vi "ABB clear results.vi"   [LabVIEW 2017]
uses:
  ABB global.vi
panel:
  # "clear tests"
types:
  T1 = cluster{"Stator R":dbl, "Stator dT":dbl, "Rotor R":dbl, "Rotor dT":dbl, "Stator Cooling curve":dbl[][], "Rotor Cooling curve":dbl[][], "Select Resistance":enum16{"Fitted zero Res.", "Selected Res.", "Entered Res."}}
  T2 = cluster{"Stator R":dbl, "Stator dT":dbl, "Rotor R":dbl, "Rotor dT":dbl, "Stator Cooling curve":dbl[][], "Rotor Cooling curve":dbl[][], "Select Resistance":enum16{"Fitted zero Res.", "Selected Res.", "Entered Res."}}[]
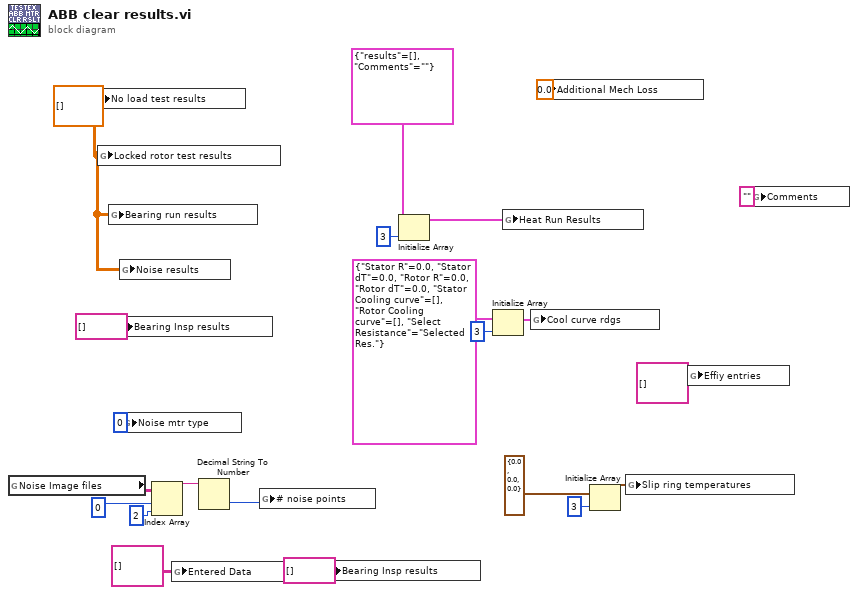
[diagram p0: block diagram]
diagram:
  w22 = dbl[][] [] ("No load test results")
  n1 = global read "ABB global.vi" "Noise Image files"() -> (w10:string[][])
  n2 = global write "ABB global.vi" "No load test results"(w22) -> ()
  n3 = global write "ABB global.vi" "Locked rotor test results"(w22) -> ()
  n4 = global write "ABB global.vi" "Bearing run results"(w22) -> ()
  n5 = global write "ABB global.vi" "Bearing Insp results"(string[] [] ("Bearing Insp results")) -> ()
  n6 = global write "ABB global.vi" "Noise results"(w22) -> ()
  n7 = global write "ABB global.vi" "Noise mtr type"(0 ("# noise points")) -> ()
  n8 = Index Array(array=w10, index (row)=0 ("disabled index (row)"), index (col)=2 ("disabled index (col)")) -> (element=w7:string)
  n9 = global write "ABB global.vi" "Entered Data"(string[][] [] ("Entered Data")) -> ()
  n10 = Decimal String To Number(string=w7) -> (number=w6:i32)  [unwired: 2 in, 1 out]
  n11 = global write "ABB global.vi" "# noise points"(w6) -> ()
  n12 = global write "ABB global.vi" "Bearing Insp results"(string[] [] ("Bearing Insp results")) -> ()
  n13 = Initialize Array(cluster{"results":dbl[][], "Comments":string} {"results"=[], "Comments"=""} ("Heat Run"), 3 ("dimension size")) -> (w20:cluster{"results":dbl[][], "Comments":string}[])
  n14 = Initialize Array(T1 {"Stator R"=0.0, "Stator dT"=0.0, "Rotor R"=0.0, "Rotor dT"=0.0, "Stator Cooling curve"=[], "Rotor Cooling curve"=[], "Select Resistance"=enum."Selected Res."} ("Cool Curve Rdgs"), 3 ("dimension size")) -> (w12:T2)
  n15 = global write "ABB global.vi" "Heat Run Results"(w20) -> ()
  n16 = global write "ABB global.vi" "Cool curve rdgs"(w12) -> ()
  n17 = global write "ABB global.vi" "Additional Mech Loss"(0.0 ("Additional Mech Loss")) -> ()
  n18 = Initialize Array(cluster{"K":dbl, "L":dbl, "M":dbl} {"K"=0.0, "L"=0.0, "M"=0.0} ("Slip Ring Temperatures (° C)"), 3 ("dimension size")) -> (w3:cluster{"K":dbl, "L":dbl, "M":dbl}[])
  n19 = global write "ABB global.vi" "Slip ring temperatures"(w3) -> ()
  n20 = global write "ABB global.vi" "Effiy entries"(string[][] [] ("Effiy entries")) -> ()
  n21 = global write "ABB global.vi" "Comments"("" ("Comments")) -> ()
